vi "Actor Core.vi"(8 "error in":errorcluster, 11 "Parent Actor in":refnum<class "Parent Actor.lvclass">) -> (0 "error out":errorcluster, 3 "Actor out":refnum<class "Actor.lvclass">)   [LabVIEW 2012, in "Parent Actor.lvclass"]
doc: "(<B>Filename</B>: Actor Framework.lvlib:Actor.lvclass:Actor Core.vi)\n\nReceives messages to the actor, reacts to them, and initiates any error handling that may shut the actor down.\n\nDescendant classes may override this VI to append parallel tasks for the actor to complete while it handles messages. Overrides use the Call Parent Method node."
uses:
  Parent Actor.lvclass
  <vilib>/ActorFramework/Actor/Actor.lvclass
  Child Actor.lvclass
  <vilib>/ActorFramework/Actor/Actor.lvclass/Actor.ctl
  <vilib>/ActorFramework/Message Enqueuer/Message Enqueuer.lvclass/Message Enqueuer.ctl
  Parent Actor.lvclass/Parent Actor.ctl
  Child Actor Messages/Get Parent State Msg/Get Parent State Msg.lvclass/Get Parent State Msg.ctl
  <vilib>/ActorFramework/Message Enqueuer/Init from Existing Queue.vi
  <vilib>/ActorFramework/Message Enqueuer/Enqueue.vi
  <vilib>/ActorFramework/Message Priority Queue/Priority Enqueue.vi
  <vilib>/ActorFramework/Message Enqueuer/Message Enqueuer.lvclass
  <vilib>/ActorFramework/Stop Msg/Stop Msg.lvclass
  Child Actor Messages/Get Parent State Msg/Get Parent State Msg.lvclass
panel:
  in  "Parent Control":bool
  out "Parent Indicator":bool
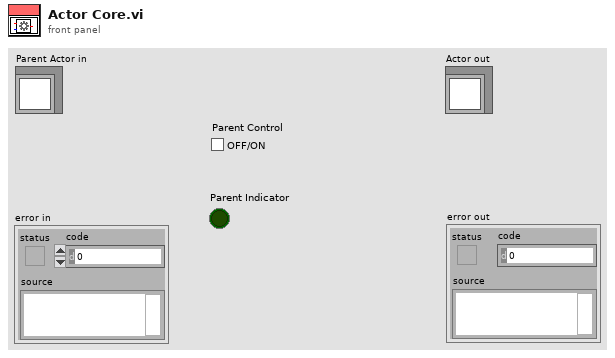
[diagram p1: front panel]
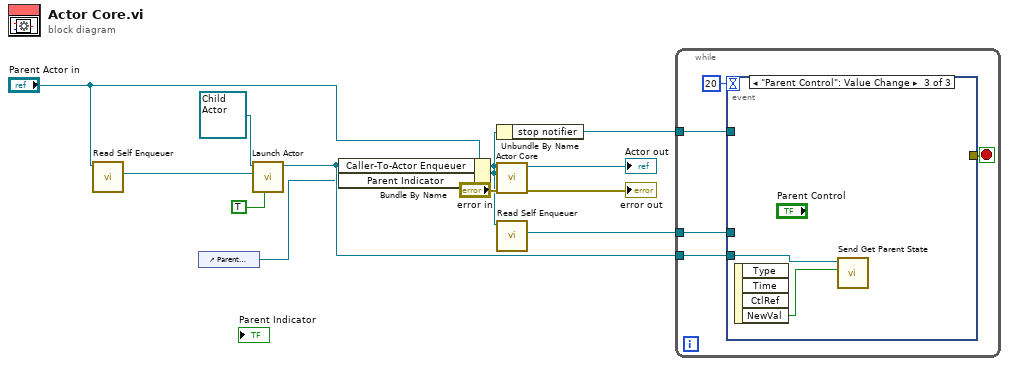
[diagram p0: block diagram]
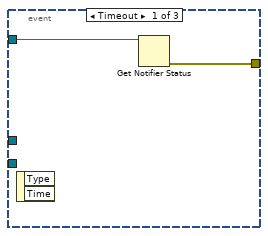
[diagram p2: hidden frame]
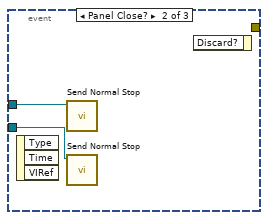
[diagram p3: hidden frame]
diagram:
  n1 = call <vilib>:"Read Self Enqueuer.vi"("Actor"="Parent Actor in") -> ("Self Enqueuer"=w8:refnum<class "Message Enqueuer.lvclass">)  [unwired: 10 in]
  n2 = control-ref of="Parent Indicator"() -> (w1:refnum<vi>)
  n3 = call <vilib>:"Launch Actor.vi"("Open Actor Core front panel? (F)"=TRUE, "Actor-to-Caller Enqueuer"=w8, "Actor"=refnum<class "Child Actor.lvclass"> refnum ("Child Actor.lvclass")) -> ("Caller-To-Actor Enqueuer"=w2:refnum<class "Message Enqueuer.lvclass">)  [unwired: 7 in, 1 out]
  n4 = Bundle By Name(cluster="Parent Actor in", "Caller-To-Actor Enqueuer"=w2, "Parent Indicator"=w1) -> (w5:refnum<class "Parent Actor.lvclass">)
  n5 = Unbundle By Name(w5) -> ("stop notifier"=w6:refnum<notifier>)
  n6 = call-parent "Actor Core.vi"("error in"="error in", "Actor in"=w5) -> ("error out"=→"error out":errorcluster, "Actor out"=→"Actor out":refnum<class "Actor.lvclass">)  [unwired: 8 in]
  n7 = call <vilib>:"Read Self Enqueuer.vi"("Actor"=w5) -> ("Self Enqueuer"=w4:refnum<class "Message Enqueuer.lvclass">)  [unwired: 10 in]
  n8 = while {
    tunnel: w6 -> [w15]
    tunnel: w4 -> [w14]
    tunnel: w2 -> [w13]
    stop <- w16 stop-if-true
    n9 = event shown="[2] \"Parent Control\": Value Change" {
      selector: _ -> [_ _ _]
      dyn-events: _ -> [_ _ _]
      timeout: 20 -> [_ _ _]
      tunnel: [w19 _ _] -> w16
      tunnel: w15 -> [w18 _ _]
      tunnel: w14 -> [_ w21 _]
      tunnel: w13 -> [_ w20 w23]
      event Timeout {
        n10 = event-data() -> ()  [unwired: 1 in, 2 out]
        n11 = Get Notifier Status(notifier=w18) -> (error out=w19:errorcluster)  [unwired: 1 in, 4 out]
      }
      event Panel Close? {
        n12 = event-data() -> ()  [unwired: 1 in, 3 out]
        n13 = call <vilib>:"Send Normal Stop.vi"("Message Enqueuer"=w21) -> ()  [unwired: 10 in, 1 out]
        n14 = call <vilib>:"Send Normal Stop.vi"("Message Enqueuer"=w20) -> ()  [unwired: 10 in, 1 out]
        n15 = event-data() -> ()  [unwired: 2 in, 1 out]
      }
      event "Parent Control": Value Change {
        n16 = event-data() -> ("NewVal"=w22:bool)  [unwired: 1 in, 3 out]
        n17 = call "Send Get Parent State.vi"("Boolean"=w22, "Message Enqueuer"=w23) -> ()  [unwired: 8 in, 2 out]
      }
    }
  }
